vi "Set Camera Mode Message to JSON.vi"(2 "error in":errorcluster, 3 "Set Camera Mode Message":T1) -> (0 "error out":errorcluster, 1 "JSON string":string)   [LabVIEW 2016]
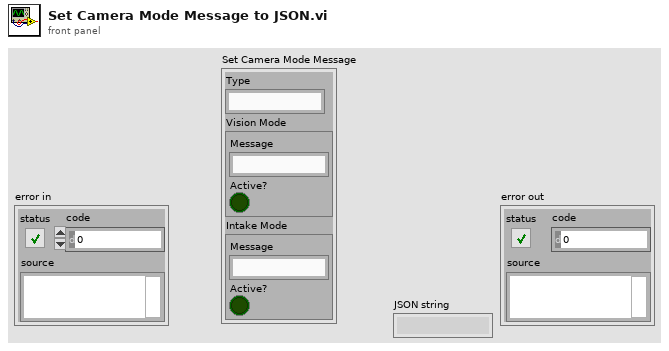
[diagram p1: front panel]
types:
  T1 = cluster{"Type":string, "Vision Mode":cluster{"Message":string, "Active?":bool}, "Intake Mode":cluster{"Message":string, "Active?":bool}}
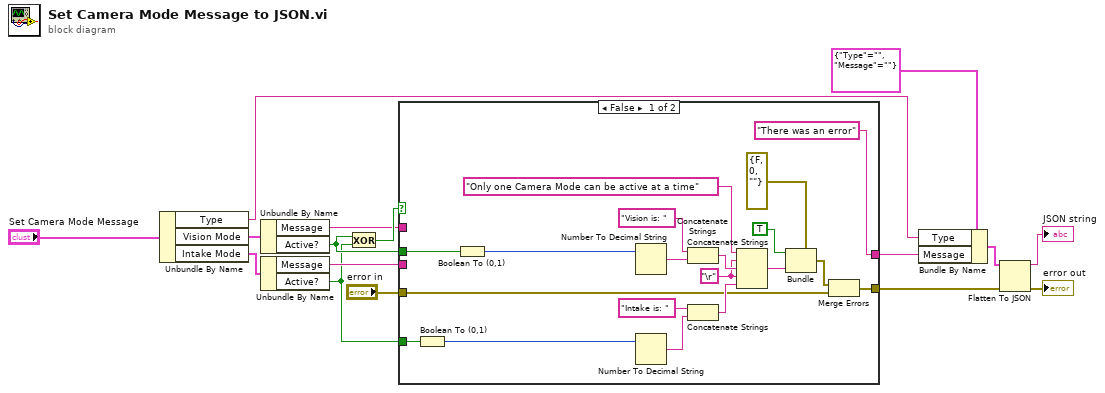
[diagram p0: block diagram]
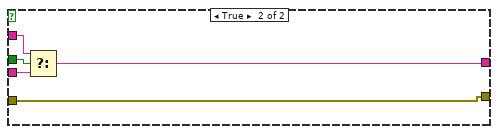
[diagram p2: hidden frame]
diagram:
  n1 = Unbundle By Name("Set Camera Mode Message") -> ("Type"=w3:string, "Vision Mode"=w13:cluster{"Message":string, "Active?":bool}, "Intake Mode"=w12:cluster{"Message":string, "Active?":bool})
  n2 = Unbundle By Name(w13) -> ("Message"=w9:string, "Active?"=w10:bool)
  n3 = Unbundle By Name(w12) -> ("Message"=w8:string, "Active?"=w7:bool)
  n4 = Exclusive Or(1:w7, 2:w10) -> (0:w11:bool)
  n5 = case shown="False" w11 {
    tunnel: w10 -> [w31 w40]
    tunnel: w9 -> [_ w39]
    tunnel: w8 -> [_ w38]
    tunnel: ["There was an error" ("Message") w37] -> w2
    tunnel: w7 -> [w24 _]
    tunnel: "error in" -> [w19 w36]
    tunnel: [w18 w36] -> w5
    frame False {
      w28 = "\r"
      n6 = Boolean To (0,1)(Boolean=w24) -> (0, 1=w25:i16)
      n7 = Boolean To (0,1)(Boolean=w31) -> (0, 1=w30:i16)
      n8 = Number To Decimal String(number=w30) -> (decimal integer string=w27:string)  [unwired: 1 in]
      n9 = Number To Decimal String(number=w25) -> (decimal integer string=w23:string)  [unwired: 1 in]
      n10 = Concatenate Strings("Vision is: " ("string"), w27) -> (w29:string)
      n11 = Concatenate Strings("Intake is: " ("string"), w23) -> (w22:string)
      n12 = Concatenate Strings("Only one Camera Mode can be active at a time" ("source"), w28, w29, w28, w22) -> (w21:string)
      n13 = Bundle(cluster=errorcluster {"status"=FALSE, "code"=0, "source"=""} ("error constant"), "status"=TRUE, "source"=w21) -> (w20:errorcluster)  [unwired: 1 in]
      n14 = Merge Errors(w20, w19) -> (w18:errorcluster)
    }
    frame True {
      n15 = Select(t=w39, s=w40, f=w38) -> (s? t:f=w37:string)
    }
  }
  n16 = Bundle By Name(cluster=cluster{"Type":string, "Message":string} {"Type"="", "Message"=""}, "Type"=w3, "Message"=w2) -> (w1:cluster{"Type":string, "Message":string})
  n17 = Flatten To JSON(anything=w1, error in (no error)=w5) -> (JSON string=→"JSON string":string, 11:→"error out":errorcluster)  [unwired: 1 in]
